vi "Close.vi"(8 "error in (no error)":errorcluster, 9 "Sample quantum (min 1)":i32=1 min=1, 10 "Dig waveform to prepend":digitalwaveform(waveform)={"t0"=timestamp(0 s since 1904-01-01), "dt"=0.0, "Y"={"transitions"=[], "data"=[]}, "error"={"status"=FALSE, "code"=37421928, "source"=""}}, 11 "I2C waveform info":T2) -> (0 "error out":errorcluster, 1 "Compare bits":cluster{"Locations":u64[], "Types":T1[]}, 2 "Dig waveform out":digitalwaveform(waveform)={"t0"=timestamp(0 s since 1904-01-01), "dt"=0.0, "Y"={"transitions"=[], "data"=[]}, "error"={"status"=FALSE, "code"=37421928, "source"=""}})   [LabVIEW 2009, in "IDW.lvlib"]
doc: "Converts an I2C waveform into a Digital Waveform Datatype (DWDT). Also optionally appends this waveform to an existing waveform. If this waveform is appended to an existing one, the values in the <b>Compare bits:Locations</b> array will be relative to the entire length of the appended waveform.\n\nIf the <b>Preallocated</b> instance of the <b>Init</b> VI was used to initialize the waveform, this VI checks to verify that the waveform components did not exceed allocated memory. If so, some components may have been lost during generation."
uses:
  IDW.lvlib
  _Typedefs/Waveform info.ctl
  _Typedefs/Timing - ticks.ctl
  _Typedefs/Default transition action.ctl
  _Typedefs/Bit type.ctl
  <vilib>/Waveform/DWDTOps.llb/DWDT Append Digital Samples.vi
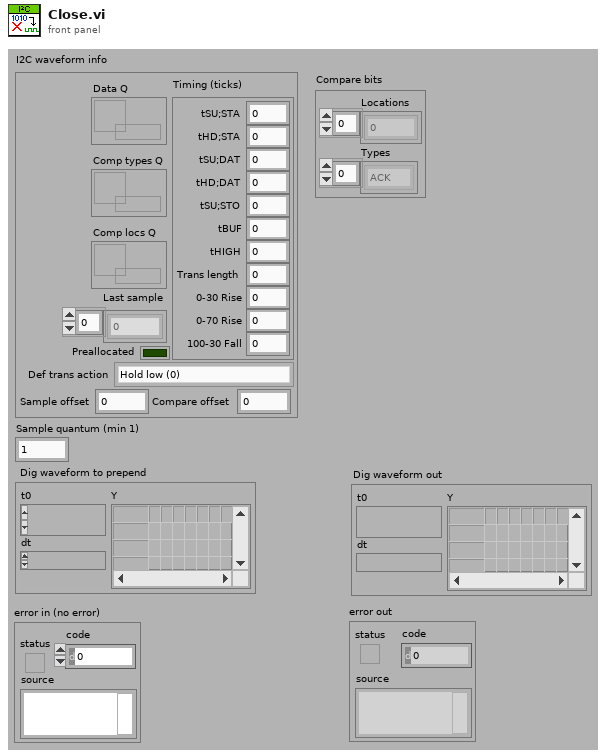
[diagram p1: front panel]
types:
  T1 = typedef "IDW.lvlib/Bit type.ctl" = enum16{"ACK", "Data"}
  T2 = typedef "IDW.lvlib/Waveform info.ctl" = cluster{"Last sample":u8[], "Sample offset":u64, "Compare offset":u64, "Timing (ticks)":T3, "Preallocated":bool, "Def trans action":T4, "Data Q":refnum<queue>, "Comp types Q":refnum<queue>, "Comp locs Q":refnum<queue>}
  T3 = typedef "IDW.lvlib/Timing - ticks.ctl" = cluster{"tSU;STA":i32, "tHD;STA":i32, "tSU;DAT":i32, "tHD;DAT":i32, "tSU;STO":i32, "tBUF":i32, "tHIGH":i32, "Trans length":i32, "0-30 Rise":i32, "0-70 Rise":i32, "100-30 Fall":i32}
  T4 = typedef "IDW.lvlib/Default transition action.ctl" = enum16{"Hold low (0)", "Release (Z)", "Set up next value", "Hold previous value", "Preserve tHD;DAT and tSU;DAT"}
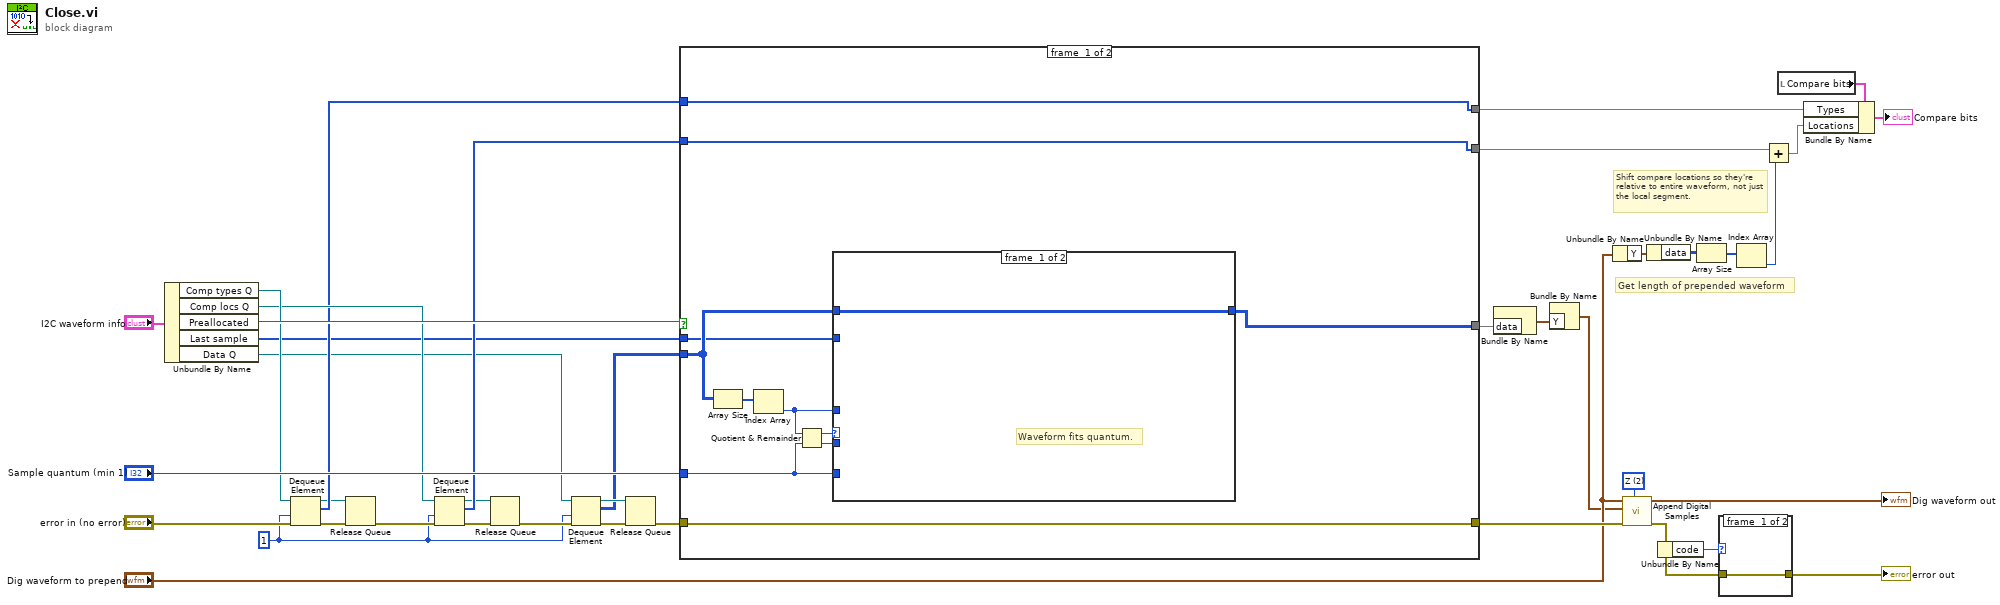
[diagram p0: block diagram]
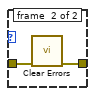
[diagram p2: hidden frame]
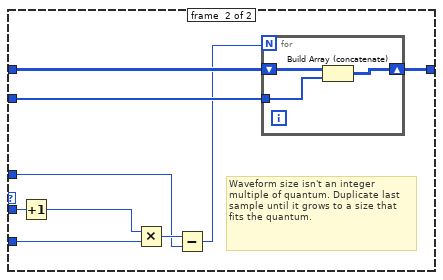
[diagram p3: hidden frame]
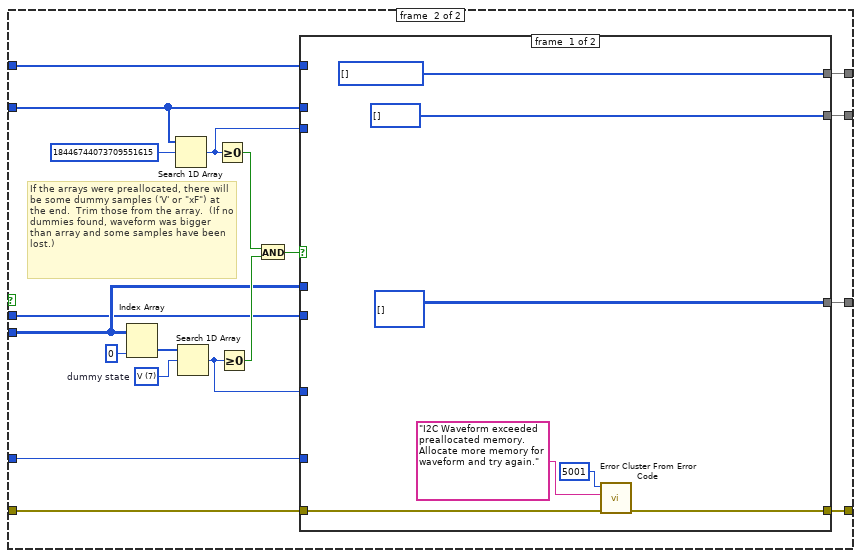
[diagram p4: hidden frame]
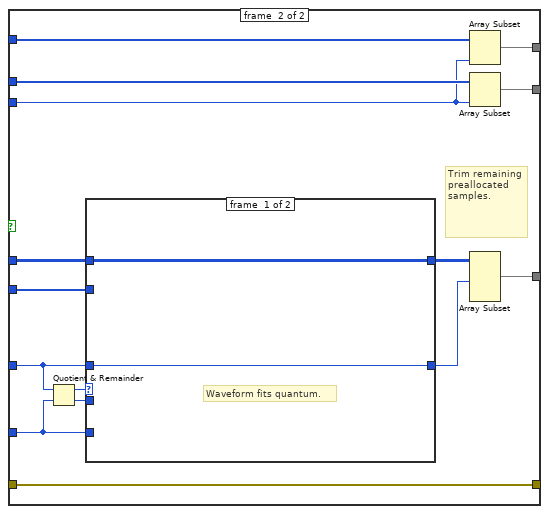
[diagram p5: hidden frame]
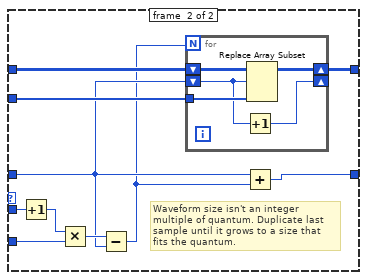
[diagram p6: hidden frame]
diagram:
  w4 = 1 ("timeout in ms (-1)")
  w39 = u8 2 items=["0", "1", "Z", "L", "H", "X", "T", "V"] ("default value")
  # "Shift compare locations so they're relative to entire waveform, not just the local segment."
  # "Get length of prepended waveform"
  n1 = Unbundle By Name("I2C waveform info") -> ("Comp types Q"=w17:refnum<queue>, "Comp locs Q"=w16:refnum<queue>, "Preallocated"=w37:bool, "Last sample"=w1:u8[], "Data Q"=w2:refnum<queue>)
  n2 = Dequeue Element(queue=w17, timeout in ms (-1)=w4, error in (no error)="error in (no error)") -> (queue out=w12:refnum<queue>, element=w14:T1[], error out=w13:errorcluster)  [unwired: 1 out]
  n3 = Release Queue(queue=w12, error in (no error)=w13) -> (error out=w5:errorcluster)  [unwired: 1 in, 2 out]
  n4 = Dequeue Element(queue=w16, timeout in ms (-1)=w4, error in (no error)=w5) -> (queue out=w10:refnum<queue>, element=w15:u64[], error out=w11:errorcluster)  [unwired: 1 out]
  n5 = Release Queue(queue=w10, error in (no error)=w11) -> (error out=w6:errorcluster)  [unwired: 1 in, 2 out]
  n6 = Dequeue Element(queue=w2, timeout in ms (-1)=w4, error in (no error)=w6) -> (queue out=w8:refnum<queue>, element=w3:u8[][], error out=w9:errorcluster)  [unwired: 1 out]
  n7 = Release Queue(queue=w8, error in (no error)=w9) -> (error out=w7:errorcluster)  [unwired: 1 in, 2 out]
  n8 = case shown="True" w37 {
    tunnel: w3 -> [w47 w80]
    tunnel: [w43 w78] -> w36
    tunnel: w7 -> [w51 w77]
    tunnel: [w51 w76] -> w35
    tunnel: "Sample quantum (min 1)" -> [w45 w74]
    tunnel: w1 -> [w46 w73]
    tunnel: w15 -> [w42 w69]
    tunnel: [w42 w67] -> w32
    tunnel: w14 -> [w41 w66]
    tunnel: [w41 w65] -> w25
    frame #0 {
      n9 = Array Size(array=w47) -> (size(s)=w48:i32[])
      n10 = Index Array(array=w48) -> (element=w44:i32)  [unwired: 1 in]
      n11 = Quotient & Remainder(x=w44, y=w45) -> (x-y*floor(x/y)=w50:i32, floor(x/y)=w49:i32)
      n12 = case shown="Default" w50 {
        tunnel: w46 -> [_ w60]
        tunnel: w47 -> [w52 w61]
        tunnel: w44 -> [_ w54]
        tunnel: [w52 w59] -> w43
        tunnel: w49 -> [_ w58]
        tunnel: w45 -> [_ w56]
        frame #0 {
          # "Waveform fits quantum."
        }
        frame #1 {
          # "Waveform size isn't an integer multiple of quantum. Duplicate last sample until it grows to a size that fits the quantum."
          n13 = Increment(x=w58) -> (x+1=w57:i32)
          n14 = Multiply(x=w57, y=w56) -> (x*y=w55:i32)
          n15 = Subtract(x=w55, y=w54) -> (x-y=w53:i32)
          n16 = for {
            N: w53 -> [_]
            tunnel: w60 -> [w62]
            shift-right: [w63] -> w59
            shift-left: w61 -> [w64]
            n17 = Build Array (concatenate)(w64, w62) -> (w63:u8[][])
          }
        }
      }
    }
    frame #1 {
      w82 = u8 7 items=["0", "1", "Z", "L", "H", "X", "T", "V"]  # dummy state
      # "If the arrays were preallocated, there will be some dummy samples ('V' or \"xF\") at the end.  Trim those from the array.  (If no dummies found, waveform was bigger than array and some samples have been lost.)"
      n18 = Index Array(array=w80, index (col)=0 ("disabled index (col)")) -> (element=w83:u8[])  [unwired: 1 in]
      n19 = Search 1D Array(1D array=w69, element=u64 18446744073709551615) -> (index of element=w68:i32)  [unwired: 1 out]
      n20 = Search 1D Array(1D array=w83, element=w82) -> (index of element=w79:i32)  [unwired: 1 out]
      n21 = Greater Or Equal To 0?(x=w68) -> (x >= 0?=w70:bool)
      n22 = Greater Or Equal To 0?(x=w79) -> (x >= 0?=w81:bool)
      n23 = And(x=w70, y=w81) -> (x .and. y?=w71:bool)
      n24 = case shown="True" w71 {
        tunnel: w80 -> [_ w101]
        tunnel: w79 -> [_ w99]
        tunnel: [u8[][] [] w105] -> w78
        tunnel: w77 -> [w89 w104]
        tunnel: [w88 w104] -> w76
        tunnel: w74 -> [_ w96]
        tunnel: w73 -> [_ w102]
        tunnel: w69 -> [_ w95]
        tunnel: w68 -> [_ w92]
        tunnel: [u64[] [] w94] -> w67
        tunnel: w66 -> [_ w93]
        tunnel: [w84 w91] -> w65
        frame #0 {
          w84 = T1[] [] items=["ACK", "Data"]
          n25 = call <vilib>:"Error Cluster From Error Code.vi"("error in (no error)"=w89, "error message (\"\")"="I2C Waveform exceeded preallocated memory. Allocate more memory for waveform and try again." ("error message (\"\")"), "error code (0)"=5001) -> ("error out"=w88:errorcluster)  [unwired: 1 in, 5 out]
        }
        frame #1 {
          # "Trim remaining preallocated samples."
          n26 = Quotient & Remainder(x=w99, y=w96) -> (x-y*floor(x/y)=w103:i32, floor(x/y)=w97:i32)
          n27 = case shown="Default" w103 {
            tunnel: w102 -> [_ w116]
            tunnel: w101 -> [w107 w117]
            tunnel: w99 -> [w106 w109]
            tunnel: [w107 w115] -> w100
            tunnel: [w106 w114] -> w98
            tunnel: w97 -> [_ w113]
            tunnel: w96 -> [_ w111]
            frame #0 {
              # "Waveform fits quantum."
            }
            frame #1 {
              # "Waveform size isn't an integer multiple of quantum. Duplicate last sample until it grows to a size that fits the quantum."
              n28 = Increment(x=w113) -> (x+1=w112:i32)
              n29 = Multiply(x=w112, y=w111) -> (x*y=w110:i32)
              n30 = Subtract(x=w110, y=w109) -> (x-y=w108:i32)
              n31 = for {
                N: w108 -> [_]
                tunnel: w116 -> [w121]
                shift-right: [w120] -> w115
                shift-left: w117 -> [w122]
                shift-right: [w118] -> _
                shift-left: w109 -> [w119]
                n32 = Increment(x=w119) -> (x+1=w118:i32)
                n33 = Replace Array Subset(array=w122, new element=w121, index (row)=w119) -> (w120:u8[][])  [unwired: 1 in]
              }
              n34 = Add(x=w109, y=w108) -> (x+y=w114:i32)
            }
          }
          n35 = Array Subset(array=w93, length=w92) -> (w91:T1[])  [unwired: 1 in]
          n36 = Array Subset(array=w95, length=w92) -> (w94:u64[])  [unwired: 1 in]
          n37 = Array Subset(array=w100, length (row)=w98) -> (w105:u8[][])  [unwired: 3 in]
        }
      }
    }
  }
  n38 = Bundle By Name("data"=w36) -> (w40:digitaldata)  [unwired: 1 out]
  n39 = Bundle By Name("Y"=w40) -> (w22:digitalwaveform)  [unwired: 1 out]
  n40 = Unbundle By Name("Dig waveform to prepend") -> ("Y"=w31:digitaldata)
  n41 = call-poly <vilib>:"Append Digital Samples.vi"("default value"=w39, "error in (no error)"=w35, "digital waveform B"=w22, "digital waveform A"="Dig waveform to prepend") -> ("error out"=w20:errorcluster, "digital waveform out"=→"Dig waveform out":digitalwaveform)  [unwired: 6 out]
  n42 = Unbundle By Name(w31) -> ("data"=w29:u8[][])
  n43 = Unbundle By Name(w20) -> ("code"=w21:i32)
  n44 = Array Size(array=w29) -> (size(s)=w28:i32[])
  n45 = case shown="1802, 1807" w21 {
    tunnel: w20 -> [w123 w125]
    tunnel: [w123 w124] -> w19
    frame #0 {
    }
    frame #1 {
      n46 = call <vilib>:"Clear Errors.vi"("error in (no error)"=w125) -> ("error out"=w124:errorcluster)  [unwired: 6 in]
    }
  }
  "error out" <- w19
  n47 = Index Array(array=w28) -> (element=w27:i32)  [unwired: 1 in]
  n48 = Add(x=w32, y=w27) -> (x+y=w24:u64[])
  n49 = local read "Compare bits"() -> (w26:cluster{"Locations":u64[], "Types":T1[]})
  n50 = Bundle By Name(cluster=w26, "Types"=w25, "Locations"=w24) -> (→"Compare bits":cluster{"Locations":u64[], "Types":T1[]})
